vi "AssertAnything.vi"(11 "Src":refnum<class "Anything.lvclass">) -> (3 "Src":refnum<class "Anything.lvclass">)   [LabVIEW 2020, in "OpenLvVision_OpenCv.lvlib"]
uses:
  OpenLvVision_OpenCv.lvlib
  Anything.lvclass
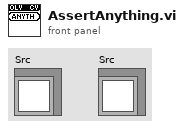
[diagram p1: front panel]
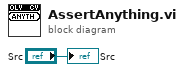
[diagram p0: block diagram]
diagram:
  "Src" <- "Src"
